vi "Camera.vi"(10 "stop":bool, 11 "Session In":T2) -> ()   [LabVIEW 2014]
uses:
  <vilib>/userdefined/High Color/IMAQdx.ctl
  <vilib>/vision/driver/NI_Vision_Acquisition_Software.lvlib
panel:
  out "Image":T1(plugin-control)
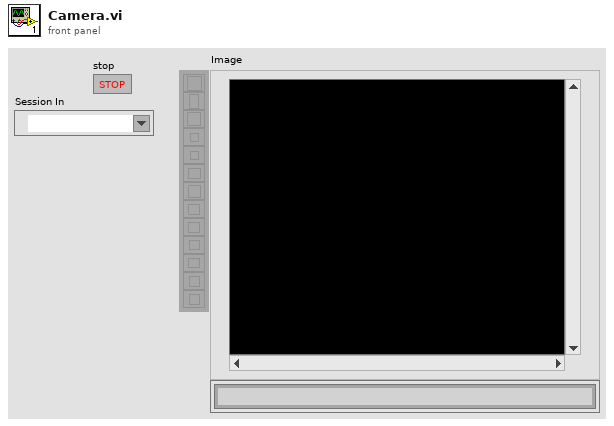
[diagram p1: front panel]
types:
  T1 = typedef "IMAQ Image.ctl" = refnum<image>
  T2 = typedef "IMAQdx.ctl" = refnum<k21>
  T3 = typedef "Image Type" = u32
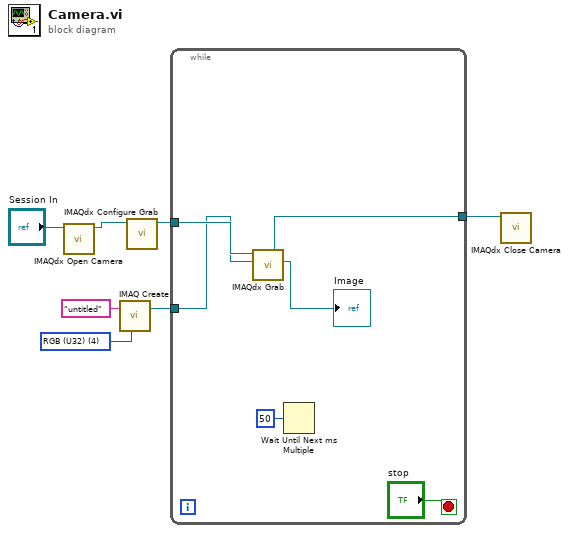
[diagram p0: block diagram]
diagram:
  w3 = T3 4 items=["Grayscale (U8)", "Grayscale (I16)", "Grayscale (SGL)", "Complex (CSG)", "RGB (U32)", "HSL (U32)", "RGB (U64)", "Grayscale (U16)"] ("Image Type")
  n1 = call <vilib>:"IMAQdx Open Camera.vi"("Session In"="Session In") -> ("Session Out"=w7:T2)  [unwired: 9 in, 1 out]
  n2 = call "IMAQ Create"("Image Name"="untitled", "Image Type"=w3) -> ("New Image"=w2:T1)  [unwired: 3 in, 1 out]
  n3 = call <vilib>:"IMAQdx Configure Grab.vi"("Session In"=w7) -> ("Session Out"=w6:T2)  [unwired: 9 in, 1 out]
  n4 = while {
    tunnel: w6 -> [w12]
    tunnel: [w11] -> w5
    tunnel: w2 -> [w10]
    stop <- "stop" stop-if-true
    n5 = call <vilib>:"IMAQdx Grab.vi"("Image In"=w10, "Session In"=w12) -> ("Image Out"=→"Image":T1, "Session Out"=w11:T2)  [unwired: 6 in, 2 out]
    n6 = Wait Until Next ms Multiple(millisecond multiple=u32 50) -> ()  [unwired: 1 out]
  }
  n7 = call <vilib>:"IMAQdx Close Camera.vi"("Session In"=w5) -> ()  [unwired: 10 in, 1 out]
